vi "conect and open C .vi"(8 "error in (no error)":errorcluster caption="错误输入（无错误）", 9 "Slot":u32, 10 "Bus":u32, 11 "Remote Machine":string="192.168.1.218") -> (0 "error out":errorcluster caption="错误输出")   [LabVIEW 2018]
uses:
  <vilib>/Utility/config.llb/Write Key (String).vi
  <vilib>/Utility/config.llb/Write Key (U32).vi
  <vilib>/Utility/config.llb/NI_LVConfig.lvlib
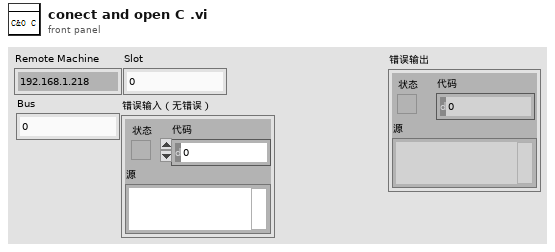
[diagram p1: front panel]
types:
  T1 = typedef "NI_LVConfig.lvlib/Config Data RefNum.ctl" = refnum<k1>
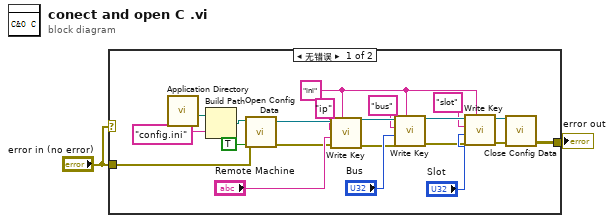
[diagram p0: block diagram]
diagram:
  n1 = case shown="无错误" "error in (no error)" {
    tunnel: "error in (no error)" -> [w6 w24]
    tunnel: [w3 w24] -> w2
    frame No Error {
      w20 = "ini" ("section")
      n2 = call <vilib>:"Application Directory.vi"() -> ("Application Directory"=w23:path)
      n3 = Build Path(base path=w23, name or relative path="config.ini" ("名称或相对路径")) -> (appended path=w21:path)
      n4 = call <vilib>:"Open Config Data.vi"("error in (no error)"=w6, "create file if necessary (T)"=TRUE, "configuration file path"=w21) -> ("error out"=w9:errorcluster, "refnum"=w19:T1)  [unwired: 6 in, 1 out]
      n5 = call-poly <vilib>:"Write Key.vi"("section"=w20, "error in (no error)"=w9, "value"="Remote Machine", "key"="ip", "refnum"=w19) -> ("error out"=w8:errorcluster, "refnum out"=w18:T1)  [unwired: 4 in, 1 out]
      n6 = call-poly <vilib>:"Write Key.vi"("section"=w20, "error in (no error)"=w8, "value"="Bus", "key"="bus", "refnum"=w18) -> ("error out"=w7:errorcluster, "refnum out"=w17:T1)  [unwired: 4 in, 1 out]
      n7 = call-poly <vilib>:"Write Key.vi"("section"=w20, "error in (no error)"=w7, "value"="Slot", "key"="slot", "refnum"=w17) -> ("error out"=w4:errorcluster, "refnum out"=w5:T1)  [unwired: 4 in, 1 out]
      n8 = call <vilib>:"Close Config Data.vi"("error in (no error)"=w4, "refnum"=w5) -> ("error out"=w3:errorcluster)  [unwired: 8 in, 1 out]
    }
    frame Error {
    }
  }
  "error out" <- w2
